vi "Lower Compress Stop.vi"(8 "error in (no error)":errorcluster, 9 "Motion.lvclass":refnum<class "Motion.lvclass">, 10 "I-O.lvclass":refnum<class "I-O.lvclass">, 11 "Pick and Place in":refnum<class "Pick and Place.lvclass">) -> (0 "error out":errorcluster, 1 "Motion.lvclass":refnum<class "Motion.lvclass">, 2 "I-O out":refnum<class "I-O.lvclass">, 3 "Pick and Place Out":refnum<class "Pick and Place.lvclass">)   [LabVIEW 2016, in "Pick and Place.lvclass"]
uses:
  Pick and Place.lvclass
  Controller/I-O/I-O.lvclass
  Controller/Motion/Motion.lvclass
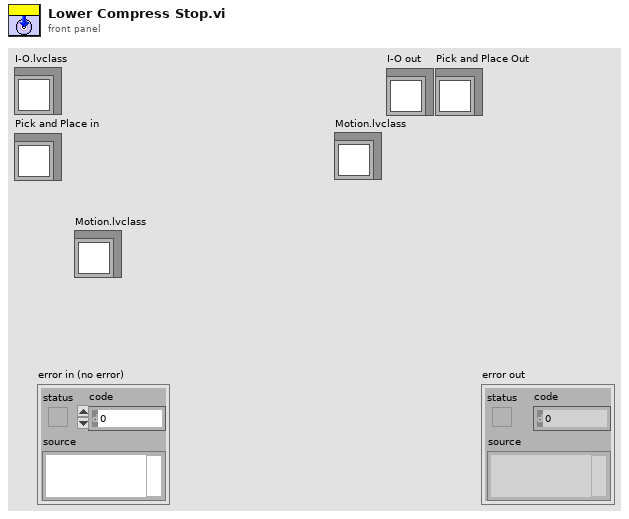
[diagram p1: front panel]
types:
  T1 = typedef "I-O.lvclass/Pin Map.ctl" = cluster{"Region Valves":i32[], "Extra Valves":dbl[][][], "Tool Primary Valve":i32, "Tool Secondary Valve":i32, "Region Sensors":i32[], "Extra Sensors":dbl[][][], "Tool Primary Sensor":dbl, "Tool Secondary Sensor":dbl, "Compression Sensor":dbl, "5V":i32}
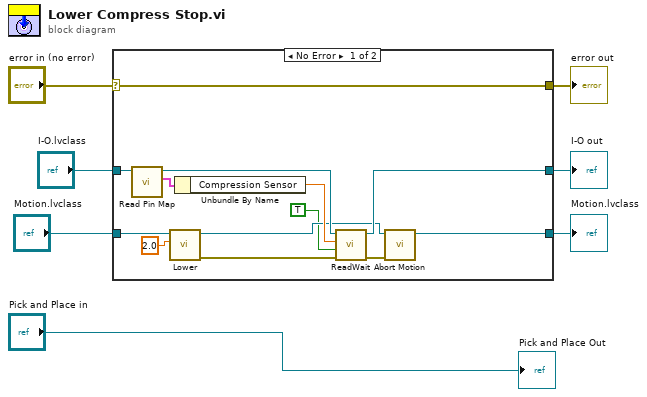
[diagram p0: block diagram]
diagram:
  n1 = case shown="No Error" "error in (no error)" {
    selector: "error in (no error)" -> [w20 w23]
    tunnel: [w20 w23] -> w6
    tunnel: "I-O.lvclass" -> [w13 w22]
    tunnel: [w17 w22] -> w4
    tunnel: [w16 w21] -> w2
    tunnel: "Motion.lvclass" -> [w15 w21]
    frame No Error {
      n2 = call-dynamic "Read Pin Map.vi"("I-O in"=w13) -> ("Pin Map 2"=w11:T1, "I-O out"=w12:refnum<class "I-O.lvclass">)  [unwired: 8 in, 1 out]
      n3 = call-dynamic "Lower.vi"("Speed"=2.0, "Motion in"=w15) -> ("error out"=w18:errorcluster, "Motion out"=w10:refnum<class "Motion.lvclass">)  [unwired: 8 in]
      n4 = Unbundle By Name(w11) -> ("Compression Sensor"=w14:dbl)
      n5 = call "ReadWait.vi"("error in (no error)"=w18, "Value"=TRUE, "Read"=w14, "I-O in"=w12) -> ("error out"=w19:errorcluster, "I-O out"=w17:refnum<class "I-O.lvclass">)  [unwired: 6 in]
      n6 = call-dynamic "Abort Motion.vi"("error in (no error)"=w19, "Motion in"=w10) -> ("Motion out"=w16:refnum<class "Motion.lvclass">)  [unwired: 8 in, 1 out]
    }
    frame Error {
    }
  }
  "error out" <- w6
  "I-O out" <- w4
  "Motion.lvclass" <- w2
  "Pick and Place Out" <- "Pick and Place in"
